vi "Initialize.vi"(8 "error in (no error)":errorcluster, 9 "Reset (True)":bool=TRUE, 10 "ID Query (True)":bool=TRUE, 11 "VISA resource name":refnum<visa-resource-name>) -> (0 "error out":errorcluster, 3 "VISA resource name out":refnum<visa-resource-name>)   [LabVIEW 2021, in "Siglent SDS 1000 2000 Series.lvlib"]
doc: "Establishes communication with the instrument and optionally performs an instrument identification query and/or an instrument reset. It also places the instrument in a default state needed for other instrument driver operations. Therefore, call this VI before calling other instrument driver VIs for this instrument. Generally, you need to call the <B>Initialize VI</B> only once at the beginning of an application."
uses:
  <instrlib>/Siglent SDS 1000 2000 Series/Siglent SDS 1000 2000 Series.lvlib
panel:
  # "(c) 2015 SIGLENT TECHNOLOGIES CO., LTD.   ALL RIGHTS RESERVED."
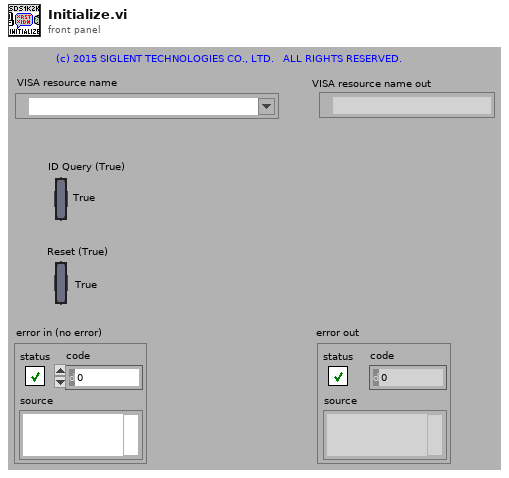
[diagram p1: front panel]
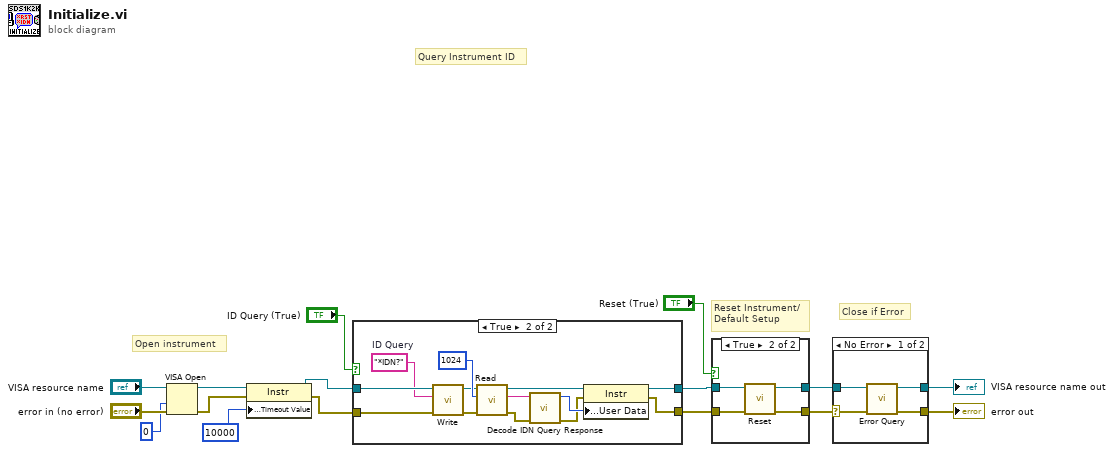
[diagram p0: block diagram]
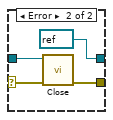
[diagram p2: hidden frame]
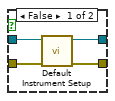
[diagram p3: hidden frame]
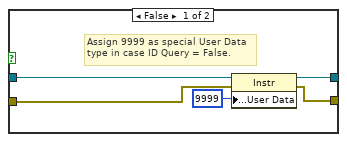
[diagram p4: hidden frame]
diagram:
  # "Close if Error"
  # "Query Instrument ID"
  # "Reset Instrument/\nDefault Setup"
  # "Open instrument"
  n1 = VISA Open(access mode=u32 0, error in (no error)="error in (no error)", VISA resource name="VISA resource name") -> (VISA resource name=w2:refnum<visa-resource-name>, error out=w1:errorcluster)  [unwired: 2 in]
  n2 = property on="Property Node" class="Instr"(reference=w2, error in=w1, "General Settings:Timeout Value"=u32 10000) -> (reference out=w5:refnum<visa-resource-name>, error out=w4:errorcluster)
  n3 = case shown="True" "ID Query (True)" {
    tunnel: [w19 w23] -> w15
    tunnel: [w18 w27] -> w16
    tunnel: w5 -> [w21 w30]
    tunnel: w4 -> [w20 w31]
    frame False {
      # "Assign 9999 as special User Data\ntype in case ID Query = False."
      n4 = property on="Property Node" class="Instr"(reference=w21, error in=w20, "General Settings:User Data"=u32 9999) -> (reference out=w18:refnum<visa-resource-name>, error out=w19:errorcluster)
    }
    frame True {
      w29 = "*IDN?"  # ID Query
      n5 = call <instrlib>:"Write.vi"("error in (no error)"=w31, "Write Buffer"=w29, "VISA resource name"=w30) -> ("error out"=w32:errorcluster, "VISA resource name out"=w33:refnum<visa-resource-name>)  [unwired: 6 in, 1 out]
      n6 = call <instrlib>:"Read.vi"("error in (no error)"=w32, "Byte Count"=u32 1024, "VISA resource name"=w33) -> ("error out"=w25:errorcluster, "Read Buffer"=w22:string, "VISA resource name out"=w28:refnum<visa-resource-name>)  [unwired: 5 in, 1 out]
      n7 = call <instrlib>:"Decode IDN Query Response.vi"("error in (no error)"=w25, "*IDN? Result"=w22) -> ("error out"=w24:errorcluster, "Series ID"=w26:u32)  [unwired: 6 in, 2 out]
      n8 = property on="Property Node" class="Instr"(reference=w28, error in=w24, "General Settings:User Data"=w26) -> (reference out=w27:refnum<visa-resource-name>, error out=w23:errorcluster)
    }
  }
  n9 = case shown="True" "Reset (True)" {
    tunnel: w15 -> [w37 w39]
    tunnel: [w36 w42] -> w6
    tunnel: w16 -> [w38 w40]
    tunnel: [w35 w41] -> w7
    frame False {
      n10 = call <instrlib>:"Default Instrument Setup.vi"("error in (no error)"=w37, "VISA resource name"=w38) -> ("error out"=w36:errorcluster, "VISA resource name out"=w35:refnum<visa-resource-name>)  [unwired: 8 in]
    }
    frame True {
      n11 = call <instrlib>:"Reset.vi"("error in (no error)"=w39, "VISA resource name"=w40) -> ("error out"=w42:errorcluster, "VISA resource name out"=w41:refnum<visa-resource-name>)  [unwired: 8 in]
    }
  }
  n12 = case shown="No Error" w6 {
    selector: w6 -> [w44 w48]
    tunnel: w7 -> [w43 w49]
    tunnel: [w46 refnum<visa-resource-name> refnum ("VISA resource name out")] -> w9
    tunnel: [w45 w50] -> w8
    frame No Error {
      n13 = call <instrlib>:"Error Query.vi"("error in (no error)"=w44, "VISA resource name"=w43) -> ("error out"=w45:errorcluster, "VISA resource name out"=w46:refnum<visa-resource-name>)  [unwired: 6 in, 2 out]
    }
    frame Error {
      n14 = call <instrlib>:"Close.vi"("error in (no error)"=w48, "VISA resource name"=w49) -> ("error out"=w50:errorcluster)  [unwired: 9 in]
    }
  }
  "VISA resource name out" <- w9
  "error out" <- w8
